vi "Aux CO2 Serial Initialize.vi"(9 "Reset CO2":bool, 11 "CO2 Channel":T4={"Serial Port"={"termination char"=10, "End read on termination character?"=TRUE, "Enabled?"=FALSE, "VISA resource name"="COM1", "baud rate"=9600, "data bits"=8, "parity"=enum."None", "stop bits"=10, "flow control"=0, "timeout (ms)"=10000, "Input buffer size"=4096, "End write on termination character?"=TRUE, "XON Char"=17, "XOFF Char"=19}, "Baro Pressure"=760, "Device"=0} {"Device" items=["None", "TidalWave", "LoFlow / Canary", "Capnogard"]; "Serial Port"."XOFF Char" format="%.0x"; "Serial Port"."XON Char" format="%.0x"; "Serial Port"."flow control" items=["None"=0, "XON/XOFF"=1, "RTS/CTS"=2, "DTR/DSR"=4]; "Serial Port"."stop bits" items=["1.0"=10, "1.5"=15, "2.0"=20]; "Serial Port"."data bits" min=5 max=8 step=1; "Serial Port"."baud rate" items=["75"=75, "110"=110, "134"=134, "150"=150, "300"=300, "600"=600, "1200"=1200, "1800"=1800, "2400"=2400, "4800"=4800, "7200"=7200, "9600"=9600, "14400"=14400, "19200"=19200, "28800"=28800, "38400"=38400, "56000"=56000, "57600"=57600, "115200"=115200, "128000"=128000, "230400"=230400]; "Serial Port"."termination char" format="%.0x"}) -> (0 "error Out":errorcluster, 1 "output cluster":T1={"Port"="", "Source"=0, "Active"=FALSE, "Baro Pressure"=760, "SerialRxBuffer"="", "Raw CO2 (Torr)"=5.0, "bytes read"=5, "Status"=[], "Status Message"=enum.""} {"Status" format="%x"; "Baro Pressure" min=400 max=800; "Source" items=["None", "TidalWave", "LoFlow / Canary", "Capnogard"]}, 2 "Serial Port Out":T3={"termination char"=10, "End read on termination character?"=TRUE, "Enabled?"=TRUE, "VISA resource name"="COM1", "baud rate"=9600, "data bits"=8, "parity"=enum."None", "stop bits"=10, "flow control"=0, "timeout (ms)"=10000, "Input buffer size"=4096, "End write on termination character?"=FALSE, "XON Char"=17, "XOFF Char"=19} {"XOFF Char" format="%.0x"; "XON Char" format="%.0x"; "flow control" items=["None"=0, "XON/XOFF"=1, "RTS/CTS"=2, "DTR/DSR"=4]; "stop bits" items=["1.0"=10, "1.5"=15, "2.0"=20]; "baud rate" items=["1.0"=10, "1.5"=15, "2.0"=20]; "termination char" format="%.0x"})   [LabVIEW 2016]
uses:
  Controls/Aux CO2 Control.ctl
  Controls/Serial Visa Control.ctl
  Controls/Aux CO2 Selector.ctl
  Controls/Aux CO2 Diags.ctl
  Controls/SerialPortControl.ctl
panel:
  # "mmHg"
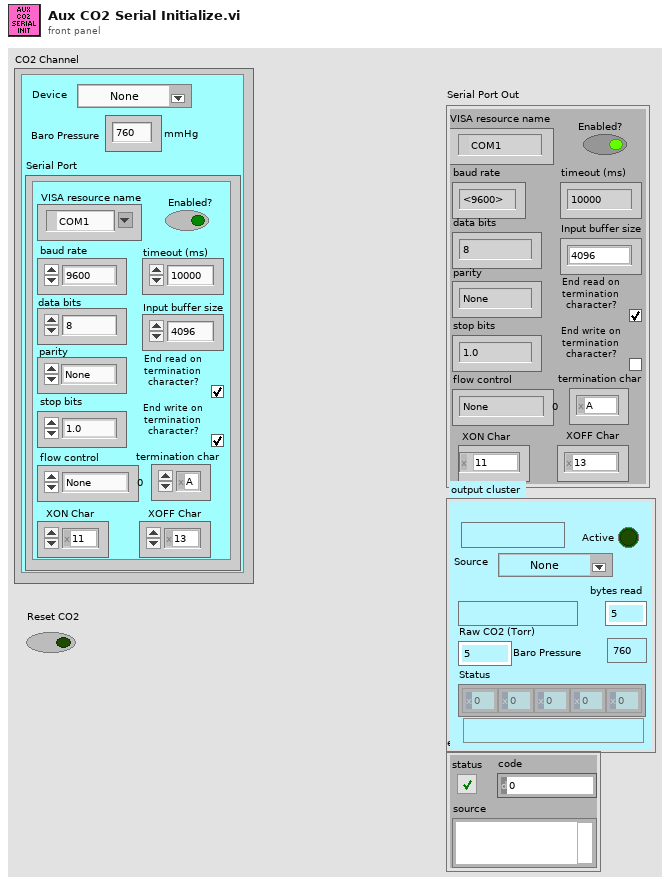
[diagram p1: front panel]
types:
  T1 = typedef "Aux CO2 Diags.ctl" = cluster{"Port":refnum<visa-resource-name>, "Source":T2, "Active":bool, "Baro Pressure":u16, "SerialRxBuffer":string, "Raw CO2 (Torr)":sgl, "bytes read":i16, "Status":u8[], "Status Message":enum16{"", "Sensor Over Temp", "Sensor Faulty", "Set BaroP", "Capno in Sleep Mode", "Zero In Progress", "Sensor Warm Up", "Check Sampling Line", "Zero Required", "CO2 Out Of Range", "Check Airway Adapter", "LoFlo Not Connected"}}
  T2 = typedef "Aux CO2 Selector.ctl" = u16
  T3 = typedef "Serial Visa Control.ctl" = cluster{"termination char":u8, "End read on termination character?":bool, "Enabled?":bool, "VISA resource name":refnum<visa-resource-name>, "baud rate":u32, "data bits":u16, "parity":enum16{"None", "Odd", "Even", "Mark", "Space"}, "stop bits":u16, "flow control":u16, "timeout (ms)":u32, "Input buffer size":u32, "End write on termination character?":bool, "XON Char":u8, "XOFF Char":u8}
  T4 = typedef "Aux CO2 Control.ctl" = cluster{"Serial Port":T3, "Baro Pressure":u32, "Device":T2}
  T5 = typedef "SerialPortControl.ctl" = enum16{"Initialize", "Write Data", "Read Data", "Close Port"}
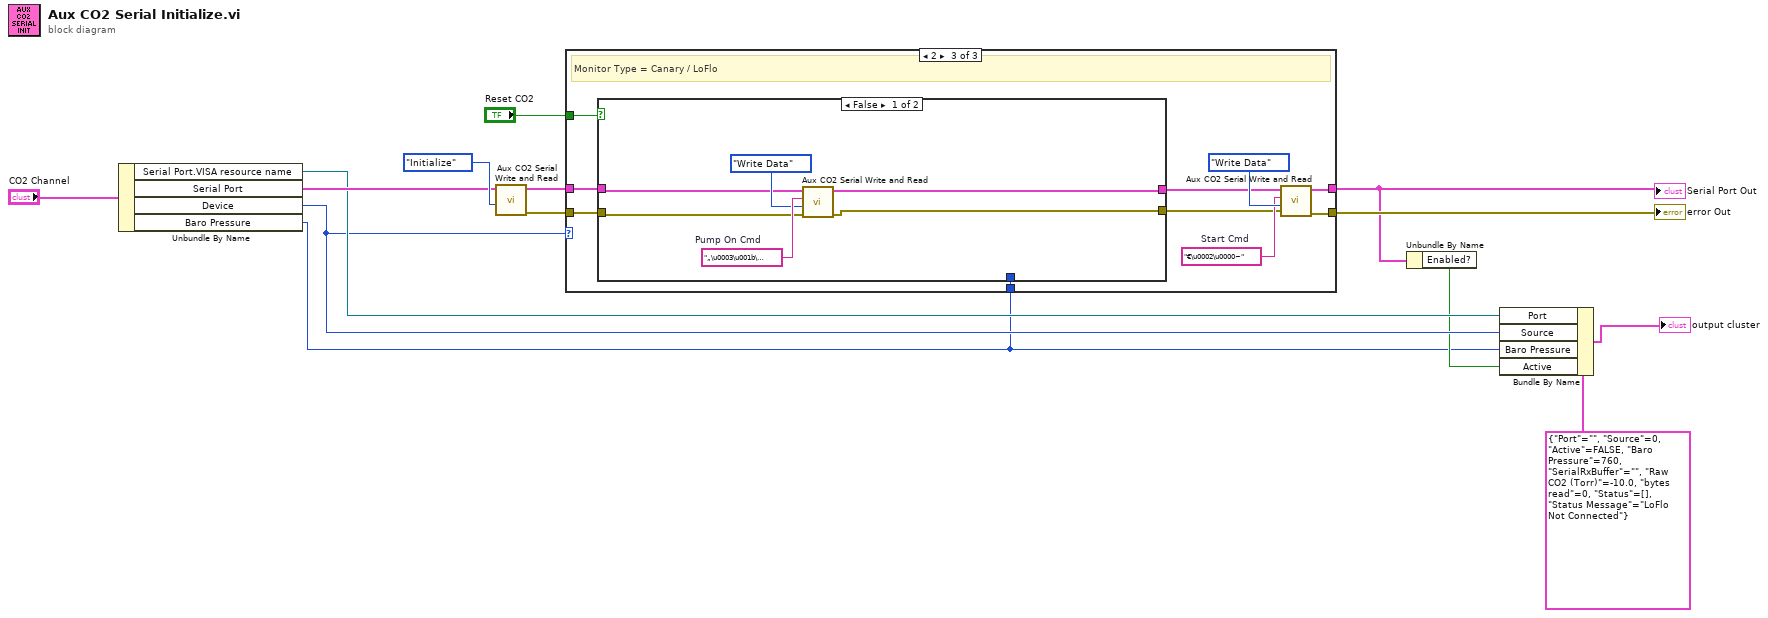
[diagram p0: block diagram]
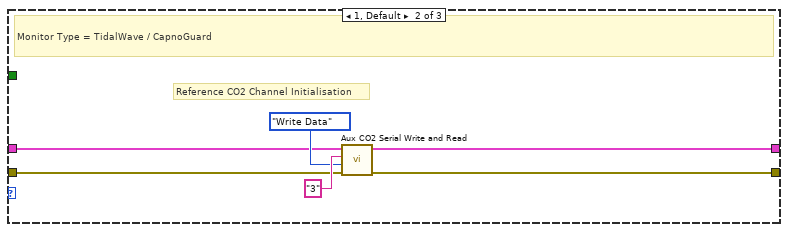
[diagram p3: hidden frame]
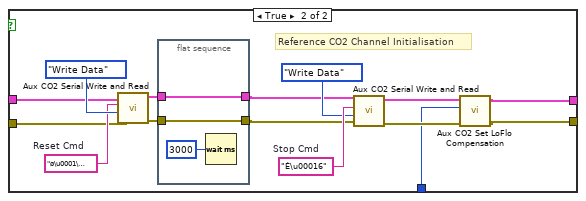
[diagram p4: hidden frame]
diagram:
  n1 = Unbundle By Name("CO2 Channel") -> ("Serial Port.VISA resource name"=w12:refnum<visa-resource-name>, "Serial Port"=w13:T3, "Device"=w7:T2, "Baro Pressure"=w2:u32)
  n2 = call "Aux CO2 Serial Write and Read.vi"("Action"=SerialPortControl."Initialize", "Serial Port"=w13) -> ("error IO"=w9:errorcluster, "Serial Port Out"=w10:T3)  [unwired: 2 in, 2 out]
  n3 = case shown="2" w7 {
    tunnel: w10 -> [w16 w17 w28]
    tunnel: [w15 w19 w30] -> w8
    tunnel: w9 -> [w15 w18 w27]
    tunnel: [w16 w20 w31] -> w6
    tunnel: w2 -> [_ _ w24]
    tunnel: "Reset CO2" -> [_ _ w23]
    frame 0 {
      # "Monitor Type = None"
    }
    frame 1, Default {
      # "Reference CO2 Channel Initialisation"
      # "Monitor Type = TidalWave / CapnoGuard"
      n4 = call "Aux CO2 Serial Write and Read.vi"("error in"=w18, "Action"=SerialPortControl."Write Data", "string to write"="3", "Serial Port"=w17) -> ("error IO"=w19:errorcluster, "Serial Port Out"=w20:T3)  [unwired: 2 out]
    }
    frame 2 {
      w29 = "€\u0002\u0000~"  # Start Cmd
      # "Monitor Type = Canary / LoFlo"
      n5 = case shown="False" w23 {
        tunnel: w28 -> [w36 w51]
        tunnel: w27 -> [w35 w50]
        tunnel: [w34 w42] -> w26
        tunnel: [w33 w41] -> w25
        tunnel: w24 -> [_ w39]
        frame False {
          w38 = "„\u0003\u001b\u0000^"  # Pump On Cmd
          n6 = call "Aux CO2 Serial Write and Read.vi"("error in"=w35, "Action"=SerialPortControl."Write Data", "string to write"=w38, "Serial Port"=w36) -> ("error IO"=w33:errorcluster, "Serial Port Out"=w34:T3)  [unwired: 2 out]
        }
        frame True {
          w47 = "É\u00016"  # Stop Cmd
          w52 = "ø\u0001\u0007"  # Reset Cmd
          # "Reference CO2 Channel Initialisation"
          n7 = call "Aux CO2 Serial Write and Read.vi"("error in"=w50, "Action"=SerialPortControl."Write Data", "string to write"=w52, "Serial Port"=w51) -> ("error IO"=w48:errorcluster, "Serial Port Out"=w49:T3)  [unwired: 2 out]
          n8 = flat-sequence {
            tunnel: [w56] -> w44
            tunnel: w49 -> [w56]
            tunnel: [w55] -> w45
            tunnel: w48 -> [w55]
            frame #0 {
              n9 = Wait (ms)(milliseconds to wait=u32 3000 ("millisecond multiple")) -> ()  [unwired: 1 out]
            }
          }
          n10 = call "Aux CO2 Serial Write and Read.vi"("error in"=w45, "Action"=SerialPortControl."Write Data", "string to write"=w47, "Serial Port"=w44) -> ("error IO"=w40:errorcluster, "Serial Port Out"=w43:T3)  [unwired: 2 out]
          n11 = call "Aux CO2 Set LoFlo Compensation.vi"("error In"=w40, "Baro Pressure"=w39, "Serial Port In"=w43) -> ("error Out"=w41:errorcluster, "Serial Port Out"=w42:T3)  [unwired: 7 in]
        }
      }
      n12 = call "Aux CO2 Serial Write and Read.vi"("error in"=w25, "Action"=SerialPortControl."Write Data", "string to write"=w29, "Serial Port"=w26) -> ("error IO"=w30:errorcluster, "Serial Port Out"=w31:T3)  [unwired: 2 out]
    }
  }
  "Serial Port Out" <- w6
  "error Out" <- w8
  n13 = Unbundle By Name(w6) -> ("Enabled?"=w5:bool)
  n14 = Bundle By Name(cluster=T1 {"Port"="", "Source"=0, "Active"=FALSE, "Baro Pressure"=760, "SerialRxBuffer"="", "Raw CO2 (Torr)"=-10.0, "bytes read"=0, "Status"=[], "Status Message"=enum."LoFlo Not Connected"} ("output cluster"), "Port"=w12, "Source"=w7, "Baro Pressure"=w2, "Active"=w5) -> (→"output cluster":T1)
